vi "Fetch Measurement (Single Point).vi"(8 "error in (no error)":errorcluster, 9 "Data Type (0: Current)":i32(ring) items=["Current", "Status", "Time", "Charge", "Humidity", "Resistance", "Source", "Temperature", "Voltage"], 10 "Channel (1: Channel 1)":i32(ring)=1 items=["Channel 1"=1], 11 "VISA resource name":refnum<visa-resource-name>) -> (0 "error out":errorcluster, 2 "Measurement":dbl, 3 "VISA resource name out":refnum<visa-resource-name>)   [LabVIEW 2017, in "Keysight B2980 Series.lvlib"]
doc: "Returns the latest voltage measurement data, current measurement data, charge measurement data, resistance measurement data, time data, status data, source output setting data, temperature data, or humidity data.\n\n<B>Note(s):</B>\nUse this VI only with other low-level VIs. The high-level VIs automatically incorporate this functionality. This VI does not check the instrument status."
uses:
  Keysight B2980 Series.lvlib
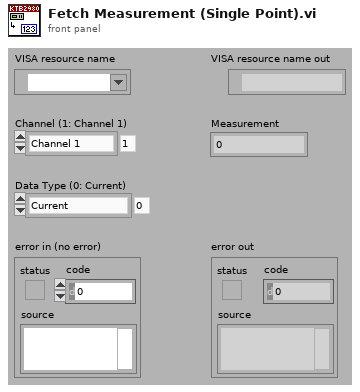
[diagram p1: front panel]
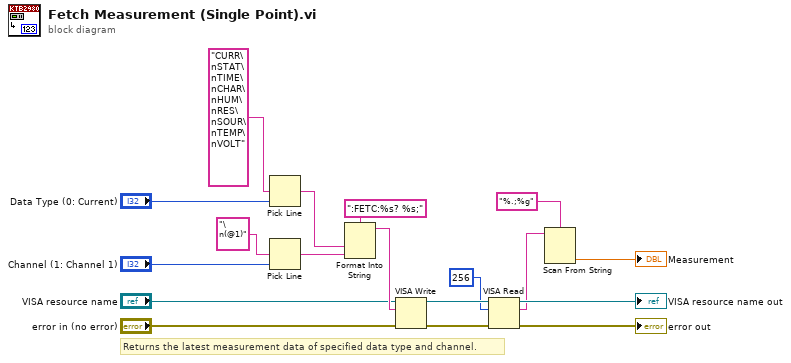
[diagram p0: block diagram]
diagram:
  # "Returns the latest measurement data of specified data type and channel."
  n1 = Pick Line(multi-line string="CURR\nSTAT\nTIME\nCHAR\nHUM\nRES\nSOUR\nTEMP\nVOLT", line index="Data Type (0: Current)") -> (output string=w15:string)  [unwired: 1 out]
  n2 = Pick Line(multi-line string="\n(@1)", line index="Channel (1: Channel 1)") -> (output string=w1:string)  [unwired: 1 out]
  n3 = Format Into String(format string=":FETC:%s? %s;", w15, w1) -> (resulting string=w14:string)  [unwired: 2 in, 1 out]
  n4 = VISA Write(VISA resource name="VISA resource name", write buffer=w14, error in (no error)="error in (no error)") -> (VISA resource name out=w11:refnum<visa-resource-name>, error out=w10:errorcluster)  [unwired: 1 out]
  n5 = VISA Read(VISA resource name=w11, byte count=u32 256, error in (no error)=w10) -> (VISA resource name out=→"VISA resource name out":refnum<visa-resource-name>, read buffer=w6:string, error out=→"error out":errorcluster)  [unwired: 1 out]
  n6 = Scan From String(format string="%.;%g", input string=w6) -> (output 1=→"Measurement":dbl)  [unwired: 2 in, 4 out]
